vi "RT_Loop.vi"(0 "PXI card names":string[](array[string])=["DIO:", "6509", "Counter:", "6733_1", "Slow AO:", "6723", "Fast AO:", "6733_1", "6733_2", "6733_3"], 1 "Param Qname":T4, 2 "RT Loop Qname":T4, 3 "Handler Qname":T4) -> ()   [LabVIEW 2018]
uses:
  <vilib>/NI/AMC/Message Queue.ctl
  <vilib>/NI/AMC/Message.ctl
  <vilib>/NI/Tools/Keyed Array/KeyedArray.ctl
  ActionCluster.ctl
  Instructions_RT.ctl
  ParameterSubCluster.ctl
  RT_State.ctl
  <vilib>/Utility/error.llb/DialogType.ctl
  Request.ctl
  <vilib>/DAQmx/read.llb/DAQmx Read (Digital 1D Bool 1Chan 1Samp).vi
  <vilib>/NI/AMC/Read Termination Message.vi
  <vilib>/NI/AMC/Create Single Message.vi
  <vilib>/NI/AMC/Update Message Routing Info.vi
  <vilib>/NI/AMC/Globals.vi
  <vilib>/NI/AMC/Send Message.vi
  <vilib>/DAQmx/miscellaneous.llb/DAQmx Fill In Error Info.vi
  <vilib>/NI/AMC/AMC.lvlib
  <vilib>/NI/Tools/Keyed Array/Tools_KeyedArray.lvlib
panel:
  in  "Consec_trigs":i32=1
  out "RT Actions":T1[](array[typedef]) {"Slow AO Array"."Duration, Gain, NewVal" format="%#_3g"}
  in  "min Action time (s)":dbl=0.01 format="%#_13g"
  in  "max Action time (s)":dbl=1000.0 format="%#_13g"
  out "error out":errorcluster
  in  "stop RT loop":bool
  out "Action #":i32=-1
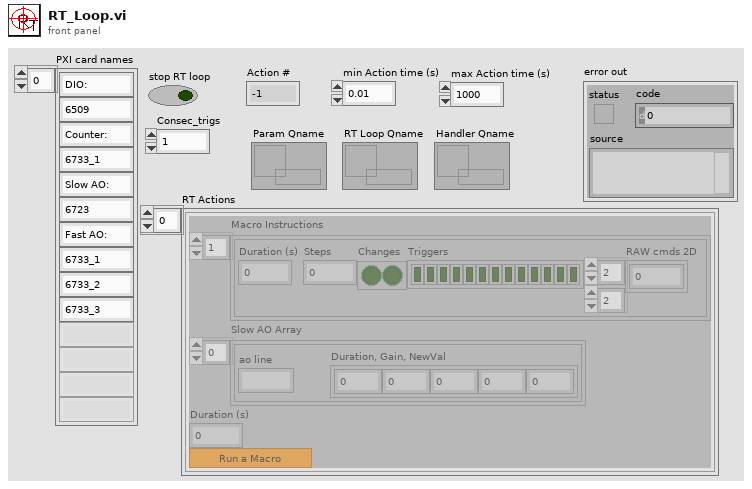
[diagram p1: front panel]
types:
  T1 = typedef "ActionCluster.ctl" = cluster{"Macro Instructions":T2, "Slow AO Array":T3, "Duration (s)":dbl, "Toggle":bool}
  T2 = typedef "Instructions_RT.ctl" = cluster{"Duration (s)":dbl, "Steps":i32, "Changes":bool[], "Triggers":bool[], "RAW cmds 2D":i16[][]}[]
  T3 = typedef "ParameterSubCluster.ctl" = cluster{"ao line":string, "Duration, Gain, NewVal":dbl[]}[]
  T4 = typedef "AMC.lvlib/Message Queue.ctl" = refnum<queue>
  T5 = typedef "DialogType.ctl" = u16
  T6 = typedef "RT_State.ctl" = enum16{"Idle", "Run", "Macro", "Param", "Inbit"}
  T7 = typedef "Tasks_RT.ctl" = cluster{"inbits":i32, "outbits":i32, "Counter":refnum<k21>, "Inbits":refnum<k21>, "Outbits":refnum<k21>, "Fast AO":refnum<k21>[], "Errors":errorcluster}
  T8 = typedef "Request.ctl" = enum16{"Start", "Run", "Skip Wait", "Pause", "Unpause", "Abort", "Shutdown"}
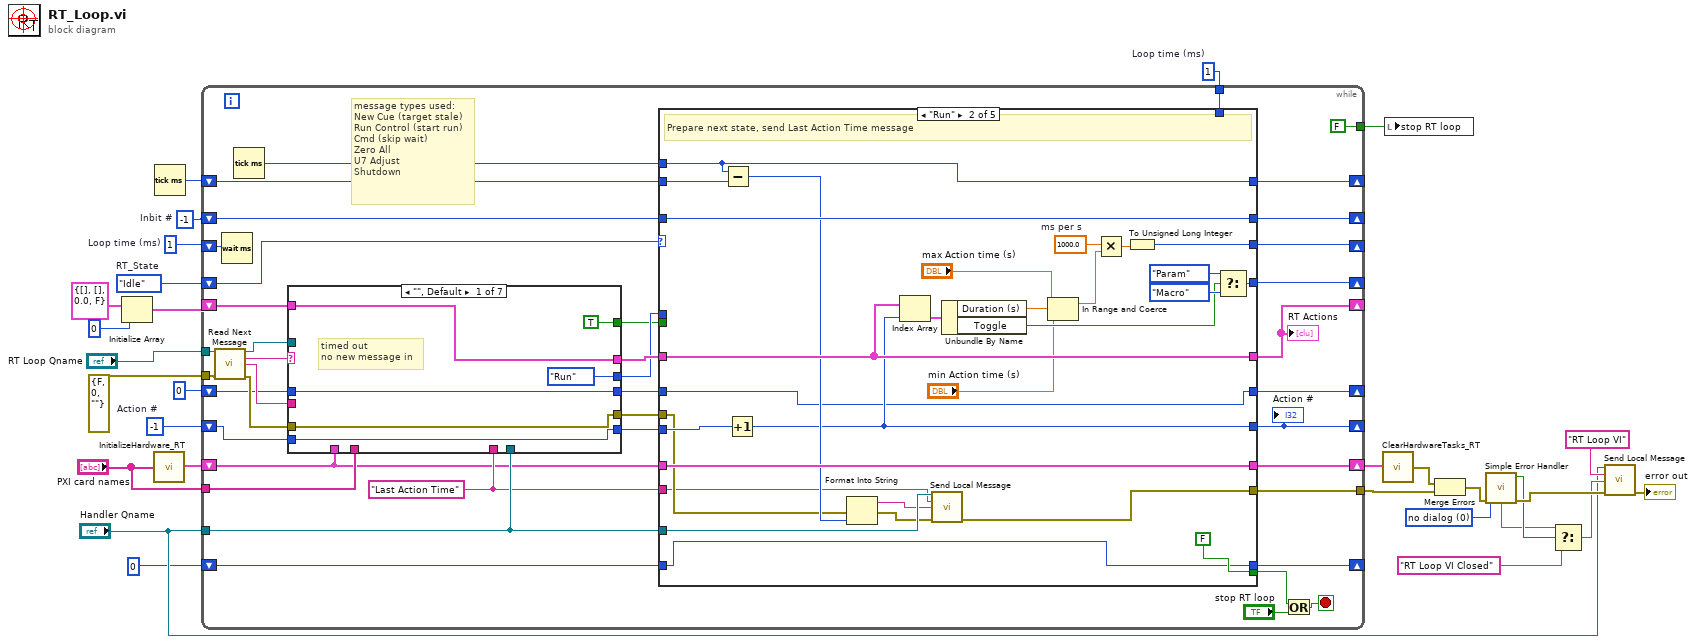
[diagram p0: block diagram]
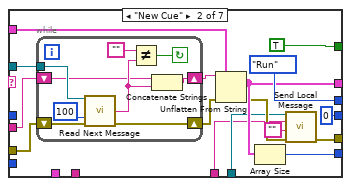
[diagram p2: hidden frame]
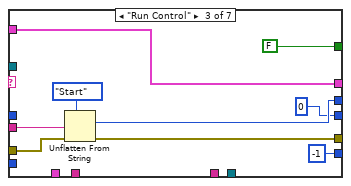
[diagram p3: hidden frame]
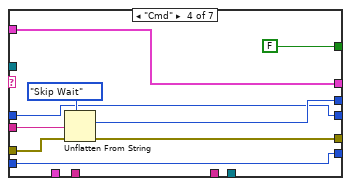
[diagram p4: hidden frame]
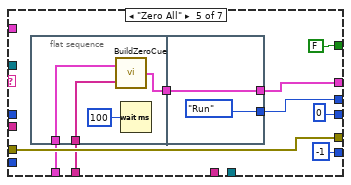
[diagram p5: hidden frame]
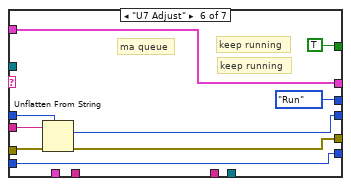
[diagram p6: hidden frame]
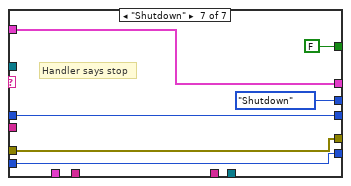
[diagram p7: hidden frame]
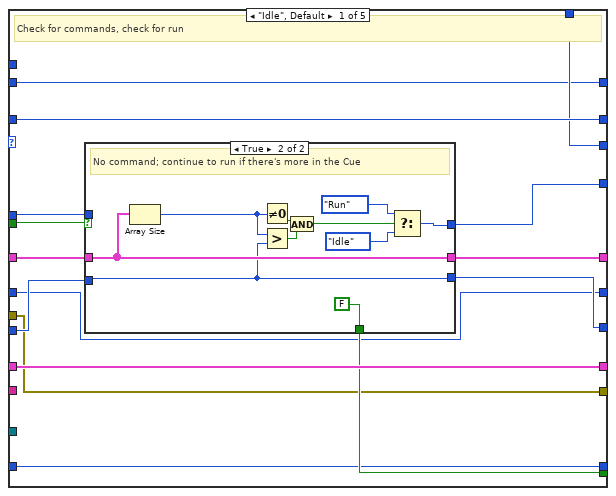
[diagram p8: hidden frame]
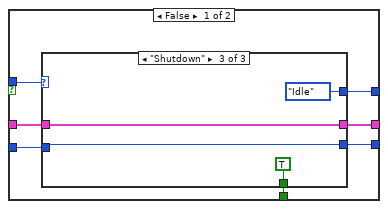
[diagram p9: hidden frame]
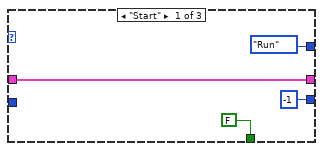
[diagram p10: hidden frame]
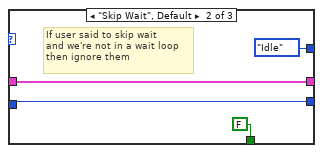
[diagram p11: hidden frame]
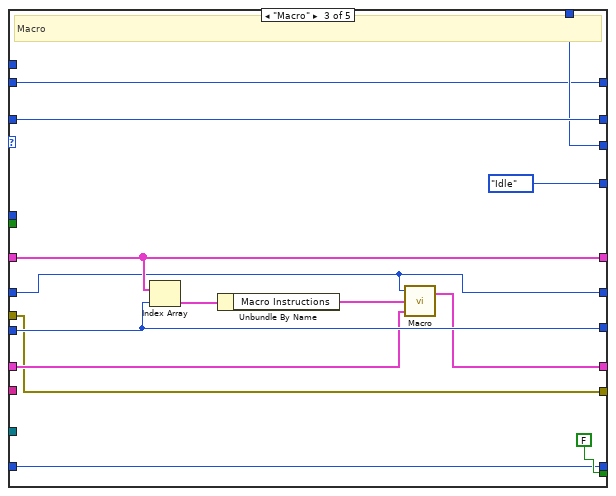
[diagram p12: hidden frame]
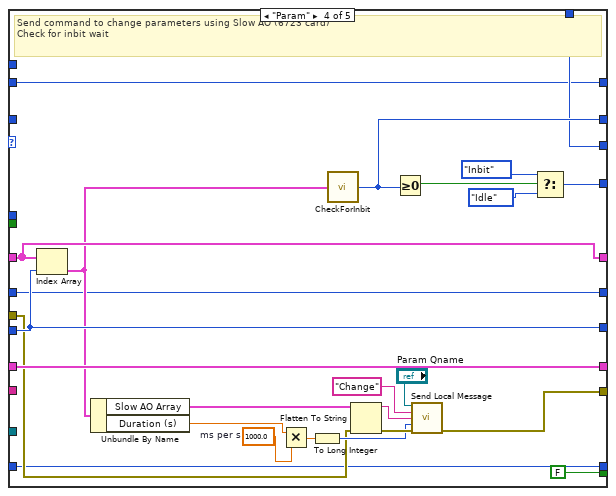
[diagram p13: hidden frame]
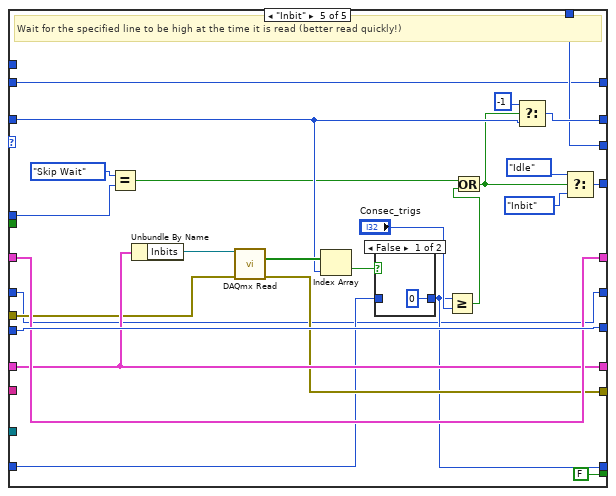
[diagram p14: hidden frame]
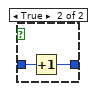
[diagram p15: hidden frame]
diagram:
  w12 = u32 1  # Loop time (ms)
  w14 = u32 1  # Loop time (ms)
  w22 = T5 0 items=["no dialog", "OK message", "continue or stop message", "OK message + warnings", "continue/stop + warnings"] ("type of dialog (OK msg:1)")
  w24 = -1  # Inbit #
  w26 = RT_State."Idle"  # RT_State
  w27 = -1  # Action #
  n1 = Initialize Array(T1 {"Macro Instructions"=[], "Slow AO Array"=[], "Duration (s)"=0.0, "Toggle"=FALSE} ("element"), 0 ("dimension size")) -> (w11:T1[])
  n2 = call "InitializeHardware_RT.vi"("PXI card names"="PXI card names") -> ("Task cluster"=w28:T7)
  n3 = Tick Count (ms)() -> (millisecond timer value=w13:u32)
  n4 = while {
    shift-right: [w68] -> _
    shift-left: w26 -> [w69]
    shift-right: [w67] -> _
    shift-left: w27 -> [w41]
    shift-right: [w66] -> _
    shift-left: w24 -> [w65]
    shift-right: [w44] -> _
    shift-left: w11 -> [w54]
    shift-right: [w64] -> w29
    shift-left: w28 -> [w36]
    shift-right: [w60] -> _
    shift-left: w14 -> [w59]
    shift-right: [w55] -> _
    shift-left: w13 -> [w56]
    tunnel: w12 -> [w58]
    tunnel: [w42] -> w10
    tunnel: "Handler Qname" -> [w39]
    tunnel: "RT Loop Qname" -> [w49]
    tunnel: errorcluster {"status"=FALSE, "code"=0, "source"=""} ("error out") -> [w48]
    tunnel: "PXI card names" -> [w37]
    shift-right: [w34] -> _
    shift-left: 0 ("dimension size") -> [w35]
    shift-right: [w31] -> _
    shift-left: i16 0 -> [w33]
    tunnel: [FALSE ("stop RT loop")] -> w1
    stop <- w63 stop-if-true
    w38 = "Last Action Time" ("message name")
    # "message types used:\nNew Cue (target stale)\nRun Control (start run)\nCmd (skip wait)\nZero All\nU7 Adjust\nShutdown"
    n5 = call <vilib>:"Read Next Message.vi"("message queue in"=w49, "error in"=w48) -> ("message queue out"=w50:T4, "message name"=w51:string, "message value"=w53:string, "error out"=w52:errorcluster)  [unwired: 6 in, 4 out]
    n6 = Wait (ms)(milliseconds to wait=w59) -> ()  [unwired: 1 out]
    n7 = Tick Count (ms)() -> (millisecond timer value=w57:u32)
    n8 = case shown="\"\", Default" w51 {
      tunnel: w53 -> [_ w85 w109 w118 _ w142 _]
      tunnel: [w72 w81 w103 w112 w126 w138 w145] -> w43
      tunnel: w52 -> [w72 w89 w108 w117 w126 w137 w145]
      tunnel: [TRUE TRUE FALSE FALSE FALSE TRUE FALSE] -> w45
      tunnel: w50 -> [_ w90 _ _ _ _ _]
      tunnel: [w70 w83 w105 w114 w125 w140 w143] -> w47
      tunnel: w54 -> [w70 w86 w105 w114 _ w140 w143]
      tunnel: [Request."Run" ("RT_State") Request."Run" ("RT_State") w104 w113 w123 Request."Run" ("RT_State") Request."Shutdown" ("RT_State")] -> w46
      tunnel: w41 -> [w71 _ _ w111 _ w136 w144]
      tunnel: [w71 w82 -1 ("Action #") w111 -1 ("Action #") w136 w144] -> w40
      tunnel: w39 -> [_ w79 _ _ _ _ _]
      tunnel: w38 -> [_ w77 _ _ _ _ _]
      tunnel: w37 -> [_ _ _ _ w121 _ _]
      tunnel: w36 -> [_ _ _ _ w120 _ _]
      tunnel: w33 -> [w73 _ _ w110 _ w135 w146]
      tunnel: [w73 i16 0 i16 0 w110 i16 0 w134 w146] -> w32
      frame "", Default {
        # "timed out\nno new message in"
      }
      frame "New Cue" {
        n9 = while {
          tunnel: w90 -> [w100]
          shift-right: [w97] -> w87
          shift-left: w89 -> [w98]
          shift-right: [w95] -> w88
          shift-left: w85 -> [w94]
          stop <- w92 continue-if-true
          n10 = call <vilib>:"Read Next Message.vi"("message queue in"=w100, "timeout (1 ms)"=100, "error in"=w98) -> ("message value"=w96:string, "error out"=w97:errorcluster)  [unwired: 5 in, 6 out]
          n11 = Not Equal?(x="", y=w96) -> (x != y?=w92:bool)
          n12 = Concatenate Strings(w94, w96) -> (w95:string)
        }
        n13 = Unflatten From String(type=w86, binary string=w88, error in (no error)=w87) -> (value=w83:T1[], error out=w80:errorcluster)  [unwired: 2 in, 1 out]
        n14 = Array Size(array=w83) -> (size(s)=w82:i32)
        n15 = call <vilib>:"Send Local Message.vi"("message queue in"=w79, "message name"=w77, "message value"="", "error in"=w80) -> ("error out"=w81:errorcluster)  [unwired: 9 in, 2 out]
      }
      frame "Run Control" {
        n16 = Unflatten From String(type=Request."Start" ("RT_State"), binary string=w109, error in (no error)=w108) -> (value=w104:T8, error out=w103:errorcluster)  [unwired: 2 in, 1 out]
      }
      frame "Cmd" {
        n17 = Unflatten From String(type=Request."Skip Wait" ("RT_State"), binary string=w118, error in (no error)=w117) -> (value=w113:T8, error out=w112:errorcluster)  [unwired: 2 in, 1 out]
      }
      frame "Zero All" {
        n18 = flat-sequence {
          tunnel: [w131] -> w124
          tunnel: w121 -> [w128]
          tunnel: w120 -> [w129]
          tunnel: [w133] -> w125
          tunnel: w124 -> [w133]
          tunnel: [Request."Run" ("RT_State")] -> w123
          frame #0 {
            n19 = call "BuildZeroCue.vi"("PXI card names"=w128, "Task cluster"=w129) -> ("Zero Cue"=w131:T1[])
            n20 = Wait (ms)(milliseconds to wait=u32 100) -> ()  [unwired: 1 out]
          }
          frame #1 {
          }
        }
      }
      frame "U7 Adjust" {
        # "keep running"
        # "ma queue"
        # "keep running"
        n21 = Unflatten From String(type=w135, binary string=w142, error in (no error)=w137) -> (value=w134:i16, error out=w138:errorcluster)  [unwired: 2 in, 1 out]
      }
      frame "Shutdown" {
        # "Handler says stop"
      }
    }
    n22 = case shown="\"Run\"" w69 {
      tunnel: [w161 w220 RT_State."Idle" ("RT_State") w257 w280] -> w68
      tunnel: [w155 w198 w226 w241 w271] -> w60
      tunnel: [w158 FALSE FALSE FALSE FALSE] -> w62
      tunnel: w47 -> [w163 w213 w231 w251 w273]
      tunnel: w40 -> [w156 w201 w233 w259 w285]
      tunnel: [w157 w202 w233 w259 w285] -> w67
      tunnel: [w162 w219 w232 w254 w276] -> w66
      tunnel: w65 -> [w162 w219 w232 _ w278]
      tunnel: [w160 w213 w231 w251 w273] -> w44
      tunnel: w36 -> [w159 w212 w230 w253 w272]
      tunnel: [w159 w212 w229 w253 w272] -> w64
      tunnel: w58 -> [w155 _ w226 w241 w271]
      tunnel: w57 -> [_ w205 _ _ _]
      tunnel: w56 -> [w152 w204 w225 w240 w270]
      tunnel: [w152 w205 w225 w240 w270] -> w55
      tunnel: w46 -> [w154 _ _ _ w267]
      tunnel: w45 -> [w153 _ _ _ _]
      tunnel: w39 -> [_ w206 _ _ _]
      tunnel: w43 -> [w151 w196 w224 w238 w269]
      tunnel: [w151 w197 w224 w239 w268] -> w42
      tunnel: w38 -> [_ w195 _ _ _]
      tunnel: w35 -> [w150 w194 w223 w237 w265]
      tunnel: [w150 w194 w223 w237 w262] -> w34
      tunnel: w32 -> [w149 w193 w222 w236 w261]
      tunnel: [w149 w193 w222 w236 w261] -> w31
      frame "Idle", Default {
        # "Check for commands, check for run"
        n23 = case shown="True" w153 {
          tunnel: w163 -> [w167 w185]
          tunnel: w156 -> [w166 w183]
          tunnel: [w169 w186] -> w161
          tunnel: w154 -> [w170 _]
          tunnel: [w168 w185] -> w160
          tunnel: [w165 FALSE] -> w158
          tunnel: [w164 w183] -> w157
          frame False {
            n24 = case shown="\"Shutdown\"" w170 {
              tunnel: [RT_State."Run" ("RT_State") RT_State."Idle" ("RT_State") RT_State."Idle" ("RT_State")] -> w169
              tunnel: [w173 w178 w181] -> w168
              tunnel: w167 -> [w173 w178 w181]
              tunnel: w166 -> [_ w175 w180]
              tunnel: [FALSE FALSE TRUE] -> w165
              tunnel: [-1 ("Action #") w175 w180] -> w164
              frame "Start" {
              }
              frame "Skip Wait", Default {
                # "If user said to skip wait\nand we're not in a wait loop\nthen ignore them"
              }
              frame "Shutdown" {
              }
            }
          }
          frame True {
            # "No command; continue to run if there's more in the Cue"
            n25 = Array Size(array=w185) -> (size(s)=w192:i32)
            n26 = Not Equal To 0?(x=w192) -> (x != 0?=w191:bool)
            n27 = Greater?(x=w192, y=w183) -> (0:w190:bool)
            n28 = And(x=w191, y=w190) -> (x .and. y?=w187:bool)
            n29 = Select(t=RT_State."Run" ("RT_State"), s=w187, f=RT_State."Idle" ("RT_State")) -> (s? t:f=w186:T6)
          }
        }
      }
      frame "Run" {
        w216 = 1000.0  # ms per s
        # "Prepare next state, send Last Action Time message"
        n30 = Subtract(x=w205, y=w204) -> (x-y=w203:u32)
        n31 = Increment(x=w201) -> (x+1=w202:i32)
        n32 = Format Into String(error in=w196, w203) -> (resulting string=w200:string, error out=w199:errorcluster)  [unwired: 2 in]
        n33 = Index Array(array=w213, index=w202) -> (element=w215:T1)
        n34 = call <vilib>:"Send Local Message.vi"("message queue in"=w206, "message name"=w195, "message value"=w200, "error in"=w199) -> ("error out"=w197:errorcluster)  [unwired: 9 in, 2 out]
        n35 = Unbundle By Name(w215) -> ("Duration (s)"=w211:dbl, "Toggle"=w214:bool)
        n36 = In Range and Coerce(upper limit="max Action time (s)", x=w211, lower limit="min Action time (s)") -> (coerced(x)=w207:dbl)  [unwired: 1 out]
        n37 = Multiply(x=w216, y=w207) -> (x*y=w208:dbl)
        n38 = To Unsigned Long Integer(number=w208) -> (unsigned 32bit integer=w198:u32)
        n39 = Select(t=RT_State."Param" ("RT_State"), s=w214, f=RT_State."Macro" ("RT_State")) -> (s? t:f=w220:T6)
      }
      frame "Macro" {
        # "Macro"
        n40 = Index Array(array=w231, index=w233) -> (element=w227:T1)
        n41 = Unbundle By Name(w227) -> ("Macro Instructions"=w228:T2)
        n42 = call "Macro.vi"("Tasks in"=w230, "Macro Instructions"=w228, "PhiCorrect_RAW"=w222) -> ("Tasks out"=w229:T7)  [unwired: 1 in]
      }
      frame "Param" {
        w244 = 1000.0  # ms per s
        # "Send command to change parameters using Slow AO (6723 card)\nCheck for inbit wait"
        n43 = Index Array(array=w251, index=w259) -> (element=w250:T1)
        n44 = Unbundle By Name(w250) -> ("Slow AO Array"=w252:T3, "Duration (s)"=w245:dbl)
        n45 = Multiply(x=w245, y=w244) -> (x*y=w243:dbl)
        n46 = To Long Integer(number=w243) -> (32bit integer=w242:i32)
        n47 = call "CheckForInbit.vi"("Action"=w250) -> ("Inbit #"=w254:i32)
        n48 = Flatten To String(anything=w252, error in (no error)=w238) -> (data string=w249:string, error out=w248:errorcluster)  [unwired: 2 in, 1 out]
        n49 = Greater Or Equal To 0?(x=w254) -> (x >= 0?=w255:bool)
        n50 = call <vilib>:"Send Local Message.vi"("message queue in"="Param Qname", "message name"="Change", "message value"=w249, "timeout (-1 ms)"=w242, "error in"=w248) -> ("error out"=w239:errorcluster)  [unwired: 8 in, 2 out]
        n51 = Select(t=RT_State."Inbit" ("RT_State"), s=w255, f=RT_State."Idle" ("RT_State")) -> (s? t:f=w257:T6)
      }
      frame "Inbit" {
        # "Wait for the specified line to be high at the time it is read (better read quickly!)"
        n52 = Equal?(x=Request."Skip Wait" ("RT_State"), y=w267) -> (x = y?=w274:bool)
        n53 = Unbundle By Name(w272) -> ("Inbits"=w284:refnum<k21>)
        n54 = call-poly <vilib>:"DAQmx Read.vi"("task/channels in"=w284, "error in"=w269) -> ("data"=w283:bool[], "error out"=w268:errorcluster)  [unwired: 11 in, 1 out]
        n55 = Index Array(array=w283, index=w278) -> (element=w266:bool)
        n56 = case shown="False" w266 {
          tunnel: w265 -> [_ w289]
          tunnel: [0 w288] -> w262
          frame False {
          }
          frame True {
            n57 = Increment(x=w289) -> (x+1=w288:i32)
          }
        }
        n58 = Greater Or Equal?(x=w262, y="Consec_trigs") -> (x >= y?=w263:bool)
        n59 = Or(x=w274, y=w263) -> (x .or. y?=w275:bool)
        n60 = Select(t=-1, s=w275, f=w278) -> (s? t:f=w276:i32)
        n61 = Select(t=RT_State."Idle" ("RT_State"), s=w275, f=RT_State."Inbit" ("RT_State")) -> (s? t:f=w280:T6)
      }
    }
    "Action #" <- w67
    "RT Actions" <- w44
    n62 = Or(x=w62, y="stop RT loop") -> (x .or. y?=w63:bool)
  }
  n63 = call "ClearHardwareTasks_RT.vi"("Task cluster"=w29) -> ("Errors"=w7:errorcluster)
  n64 = local write "stop RT loop"(w1) -> ()
  n65 = Merge Errors(w7, w10) -> (w23:errorcluster)
  n66 = call <vilib>:"Simple Error Handler.vi"("type of dialog (OK msg:1)"=w22, "error in (no error)"=w23) -> ("error?"=w19:bool, "error out"=w21:errorcluster, "message"=w18:string)  [unwired: 3 in, 2 out]
  n67 = Select(t=w18, s=w19, f="RT Loop VI Closed" ("message name")) -> (s? t:f=w17:string)
  n68 = call <vilib>:"Send Local Message.vi"("message queue in"="Handler Qname", "message name"="RT Loop VI", "message value"=w17, "error in"=w21) -> ("error out"=→"error out":errorcluster)  [unwired: 9 in, 2 out]
